vi "Update Elevator Location.vi"(8 "error in (no error)":errorcluster, 10 "Floor":T1, 11 "Sim Display Console Actor in":refnum<class "Sim Display Console Actor.lvclass">) -> (0 "error out":errorcluster, 3 "Sim Display Console Actor out":refnum<class "Sim Display Console Actor.lvclass">)   [LabVIEW 2019]
uses:
  Elevator Controller/Elevator Controller Actor Messages/Set Elevator Position from Location Msg/Set Elevator Position from Location Msg.lvclass
  <vilib>/ActorFramework/Actor/Actor.lvclass
  Sim Display Console Actor.lvclass
  C:/Workspace/CLA/Elevator AF 2nd/Dsiplay Console Actor/Dsiplay Console Actor/Dsiplay Console Actor.lvclass
  C:/Program Files (x86)/National Instruments/LabVIEW 2019/vi.lib/ActorFramework/Actor/Actor.lvclass
  Floor -Enum.ctl
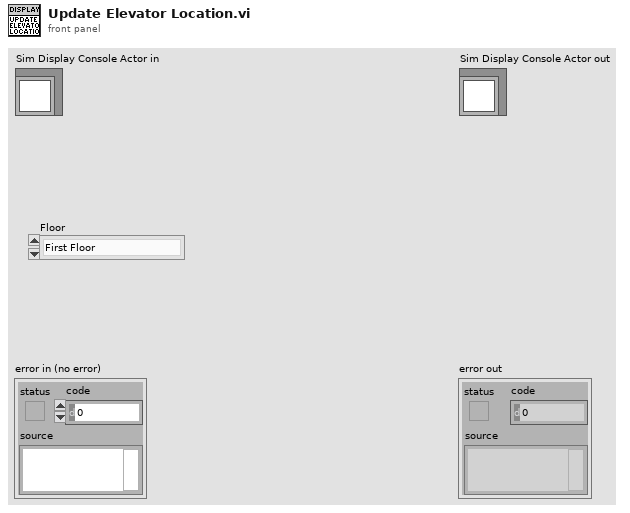
[diagram p1: front panel]
types:
  T1 = typedef "Simulated Display Console Actor.lvlib/Sim Display Console Actor.lvclass/Floor -Enum.ctl" = enum16{"First Floor", "Send Floor", "Third Floor", "Fourth Floor"}
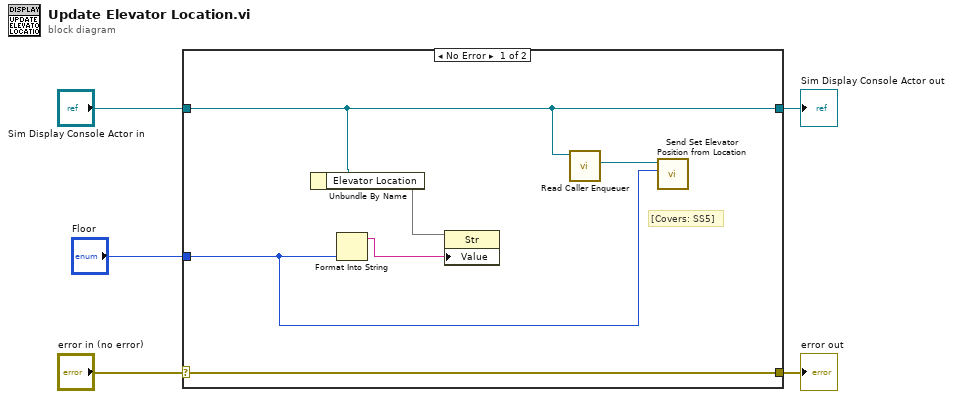
[diagram p0: block diagram]
diagram:
  n1 = case shown="No Error" "error in (no error)" {
    selector: "error in (no error)" -> [w11 w13]
    tunnel: [w11 w13] -> w4
    tunnel: [w8 w12] -> w2
    tunnel: "Sim Display Console Actor in" -> [w8 w12]
    tunnel: "Floor" -> [w6 _]
    frame No Error {
      # "[Covers: SS5]"
      n2 = Unbundle By Name(w8) -> ("Elevator Location"=w10)
      n3 = Format Into String(w6) -> (resulting string=w9:string)  [unwired: 3 in, 1 out]
      n4 = property class="Str"(reference=w10, "Value"=w9) -> ()  [unwired: 1 in, 2 out]
      n5 = call <vilib>:"Read Caller Enqueuer.vi"("Actor"=w8) -> ("Caller Enqueuer"=w7:refnum<class "Message Enqueuer.lvclass">)  [unwired: 10 in]
      n6 = call "Send Set Elevator Position from Location.vi"("Elevator Position"=w6, "Message Enqueuer"=w7) -> ()  [unwired: 8 in, 2 out]
    }
    frame Error {
    }
  }
  "error out" <- w4
  "Sim Display Console Actor out" <- w2
